vi "DSF.Shared.Configuration.Transfer Group.Set Name.vi"(8 "error in (no error)":errorcluster, 10 "Name":string, 11 "Transfer Group Configuration in":refnum<class "DSF.Shared.Configuration.Transfer Group.lvclass">) -> (0 "error out":errorcluster, 3 "Transfer Group Configuration out":refnum<class "DSF.Shared.Configuration.Transfer Group.lvclass">)   [LabVIEW 2016, in "DSF.Shared.lvlib" / "DSF.Shared.Configuration.Transfer Group.lvclass"]
uses:
  DSF.Shared.Configuration.Transfer Group.lvclass
  DSF.Shared.Configuration.Transfer Group.lvclass/DSF.Shared.Configuration.Transfer Group.ctl
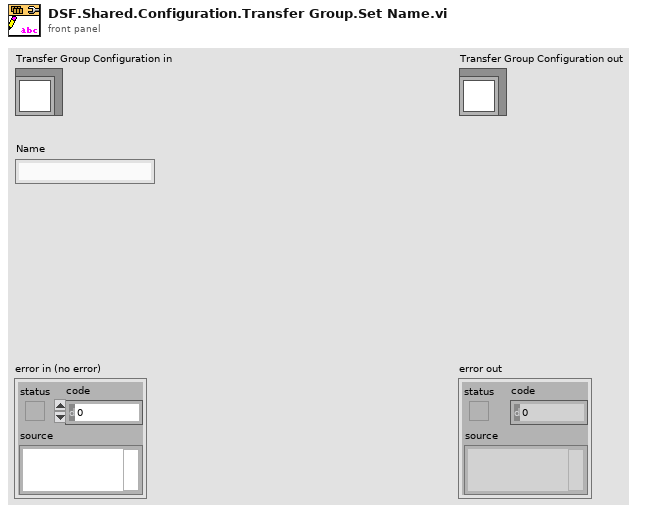
[diagram p1: front panel]
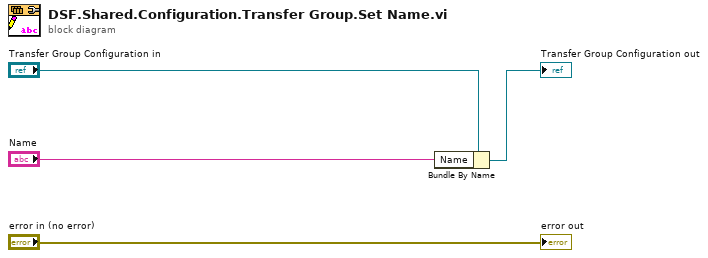
[diagram p0: block diagram]
diagram:
  n1 = Bundle By Name(cluster="Transfer Group Configuration in", "Name"="Name") -> (→"Transfer Group Configuration out":refnum<class "DSF.Shared.Configuration.Transfer Group.lvclass">)
  "error out" <- "error in (no error)"
